vi "Refresh Principal references.vi"(8 "error in":errorcluster, 11 "Project in":refnum<class "Project.lvclass">) -> (0 "error out":errorcluster, 3 "Project out":refnum<class "Project.lvclass">)   [LabVIEW 2020, in "Panther Dashboard.lvlib"]
uses:
  Panther Dashboard.lvlib
  Panther Dashboard--global.vi
  Class/Project/Project.lvclass
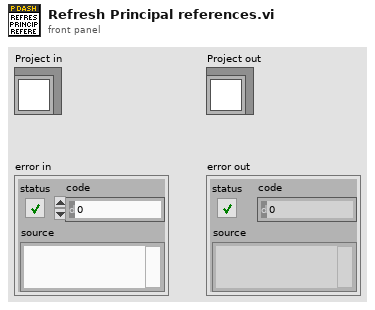
[diagram p1: front panel]
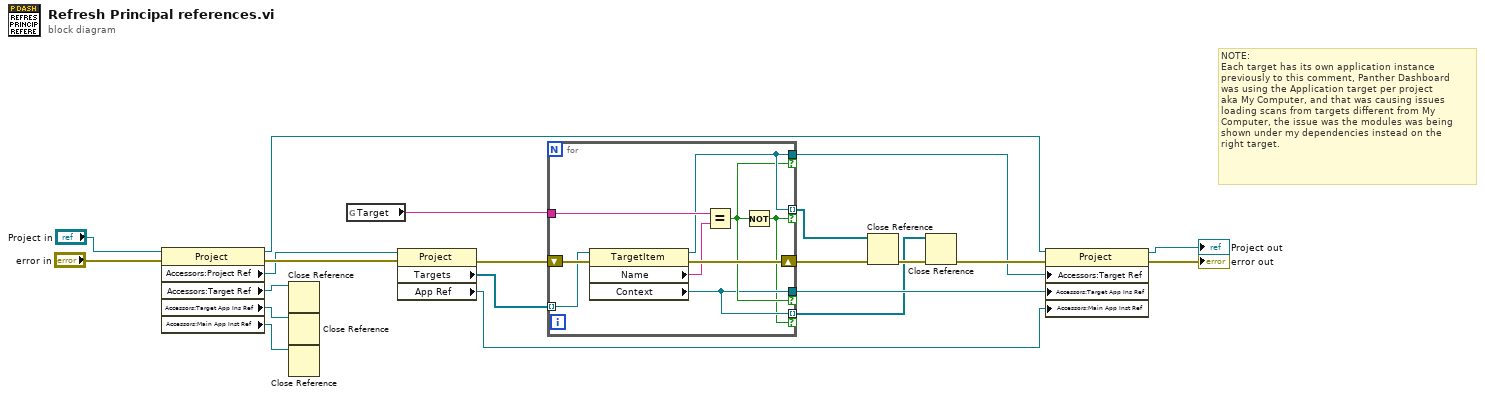
[diagram p0: block diagram]
diagram:
  # "NOTE:\nEach target has its own application instance\npreviously to this comment, Panther Dashboard\nwas using the Application target per project \naka My Computer, and that was causing issues \nloading scans from targets different from My\nComputer, the issue was the modules was being\nshown under my dependencies instead on the\nright target."
  n1 = property class="Project"(reference="Project in", error in="error in") -> (reference out=w1:refnum<class "Project.lvclass">, error out=w15:errorcluster, "Accessors:Project Ref"=w5:refnum<vi>, "Accessors:Target Ref"=w4:refnum<vi>, "Accessors:Target App Ins Ref"=w3:refnum<vi>, "Accessors:Main App Inst Ref"=w2:refnum<vi>)
  n2 = Close Reference(reference=w4) -> ()  [unwired: 1 in, 1 out]
  n3 = Close Reference(reference=w3) -> ()  [unwired: 1 in, 1 out]
  n4 = Close Reference(reference=w2) -> ()  [unwired: 1 in, 1 out]
  n5 = global read "Panther Dashboard--global.vi" "Target"() -> (w13:string)
  n6 = property class="Project"(reference=w5, error in=w15) -> (error out=w17:errorcluster, "Targets"=w8:refnum<vi>[], "App Ref"=w12:refnum<vi>)  [unwired: 1 out]
  n7 = for {
    tunnel: w8 -> [w28] mode=indexing
    tunnel: w13 -> [w26]
    tunnel: [w25] -> w10 if=w24
    tunnel: [w25] -> w7 mode=indexing if=w22
    shift-right: [w29] -> w18
    shift-left: w17 -> [w30]
    tunnel: [w23] -> w11 if=w24
    tunnel: [w23] -> w9 mode=indexing if=w22
    n8 = property class="TargetItem"(reference=w28, error in=w30) -> (reference out=w25:refnum<vi>, error out=w29:errorcluster, "Name"=w27:string, "Context"=w23:refnum<vi>)
    n9 = Equal?(x=w26, y=w27) -> (x = y?=w24:bool)
    n10 = Not(x=w24) -> (.not. x?=w22:bool)
  }
  n11 = Close Reference(reference=w7, error in (no error)=w18) -> (error out=w16:errorcluster)
  n12 = Close Reference(reference=w9, error in (no error)=w16) -> (error out=w19:errorcluster)
  n13 = property class="Project"(reference=w1, error in=w19, "Accessors:Target Ref"=w10, "Accessors:Target App Ins Ref"=w11, "Accessors:Main App Inst Ref"=w12) -> (reference out=→"Project out":refnum<class "Project.lvclass">, error out=→"error out":errorcluster)
